vi "剖面路径规划.vi"(8 "剖面底层最小深度设定":dbl, 9 "剖面单层深度设置":dbl, 10 "剖面第一层位置设定":dbl, 11 "水深":dbl) -> (1 "层数":i32, 2 "最深位置":dbl, 3 "剖面路径":dbl[](array[numeric]))   [LabVIEW 2016, in "main.lvlib"]
uses:
  main.lvlib
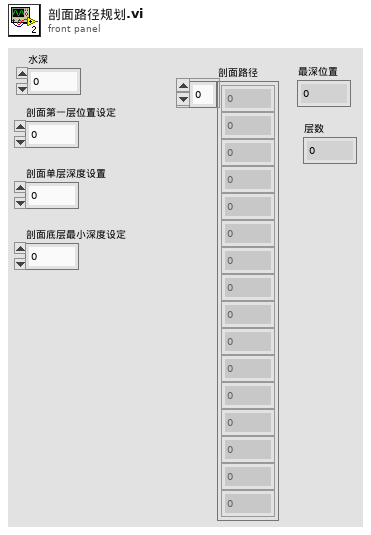
[diagram p1: front panel]
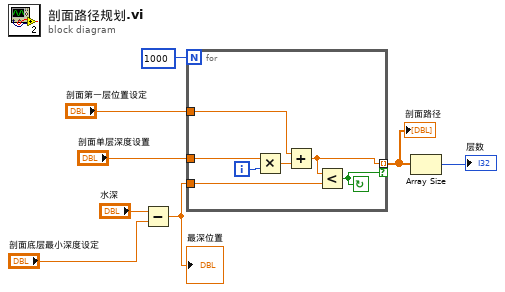
[diagram p0: block diagram]
diagram:
  n1 = Subtract(x="水深", y="剖面底层最小深度设定") -> (x-y=w8:dbl)
  "最深位置" <- w8
  n2 = for {
    N: 1000 -> [_]
    tunnel: "剖面单层深度设置" -> [w11]
    tunnel: [w9] -> w2 mode=indexing if=w13
    tunnel: w8 -> [w14]
    tunnel: "剖面第一层位置设定" -> [w15]
    i -> [w12]
    stop <- w13 continue-if-true
    n3 = Multiply(x=w11, y=w12) -> (x*y=w10:dbl)
    n4 = Add(x=w15, y=w10) -> (x+y=w9:dbl)
    n5 = Less?(x=w9, y=w14) -> (x < y?=w13:bool)
  }
  "剖面路径" <- w2
  n6 = Array Size(array=w2) -> (size(s)=→"层数":i32)
